vi "Read Waveform Channel(Single).vi"(7 "Timeout":i32=5000, 8 "error in (no error)":errorcluster, 11 "Waveform path in":string) -> (0 "error out":errorcluster, 2 "Waveform data":waveform(dbl), 3 "Waveform path out":string)   [LabVIEW 2019, in "DMA Channels Basic Testing.lvclass"]
uses:
  DMA Channels Basic Testing.lvclass
  <vilib>/NI VeriStand/Execution/WaveformStreaming/Set Rate for Waveform Stream (Acquisition Rate).vi
  <vilib>/NI VeriStand/Execution/WaveformStreaming/Set Condition for Waveform Stream (All Data).vi
  <vilib>/NI VeriStand/Execution/WaveformStreaming/Register for Waveform Data Events (DBL).vi
  <vilib>/NI VeriStand/Execution/WaveformStreaming/Unregister for Waveform Data Events (DBL).vi
  <vilib>/NI VeriStand/Execution/WaveformStreaming/NI_VS Waveform Streaming Interface.lvlib
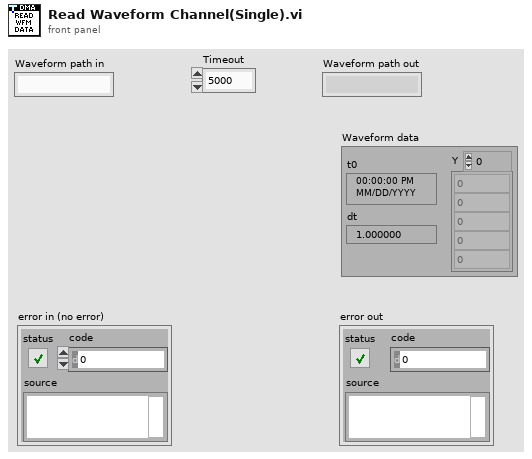
[diagram p1: front panel]
types:
  T1 = typedef "NI_VS Waveform Streaming Interface.lvlib/WaveformStreamSpecification.ctl" = refnum<k24>
  T2 = typedef "NI_VS Waveform Streaming Interface.lvlib/WaveformStreamingAPI.ctl" = refnum<k24>
  T3 = typedef "NI_VS Waveform Streaming Interface.lvlib/Registered Waveform Streams Data Event Refnum (DBL).ctl" = cluster{"Callback Refnum":refnum<k27>, "Data Event":refnum<user-event>, "Event Refnum":refnum<event-registration>, "WaveformDataWatcherDBL":T4}
  T4 = typedef "NI_VS Waveform Streaming Interface.lvlib/WaveformDataWatcherDBL.ctl" = refnum<k24>
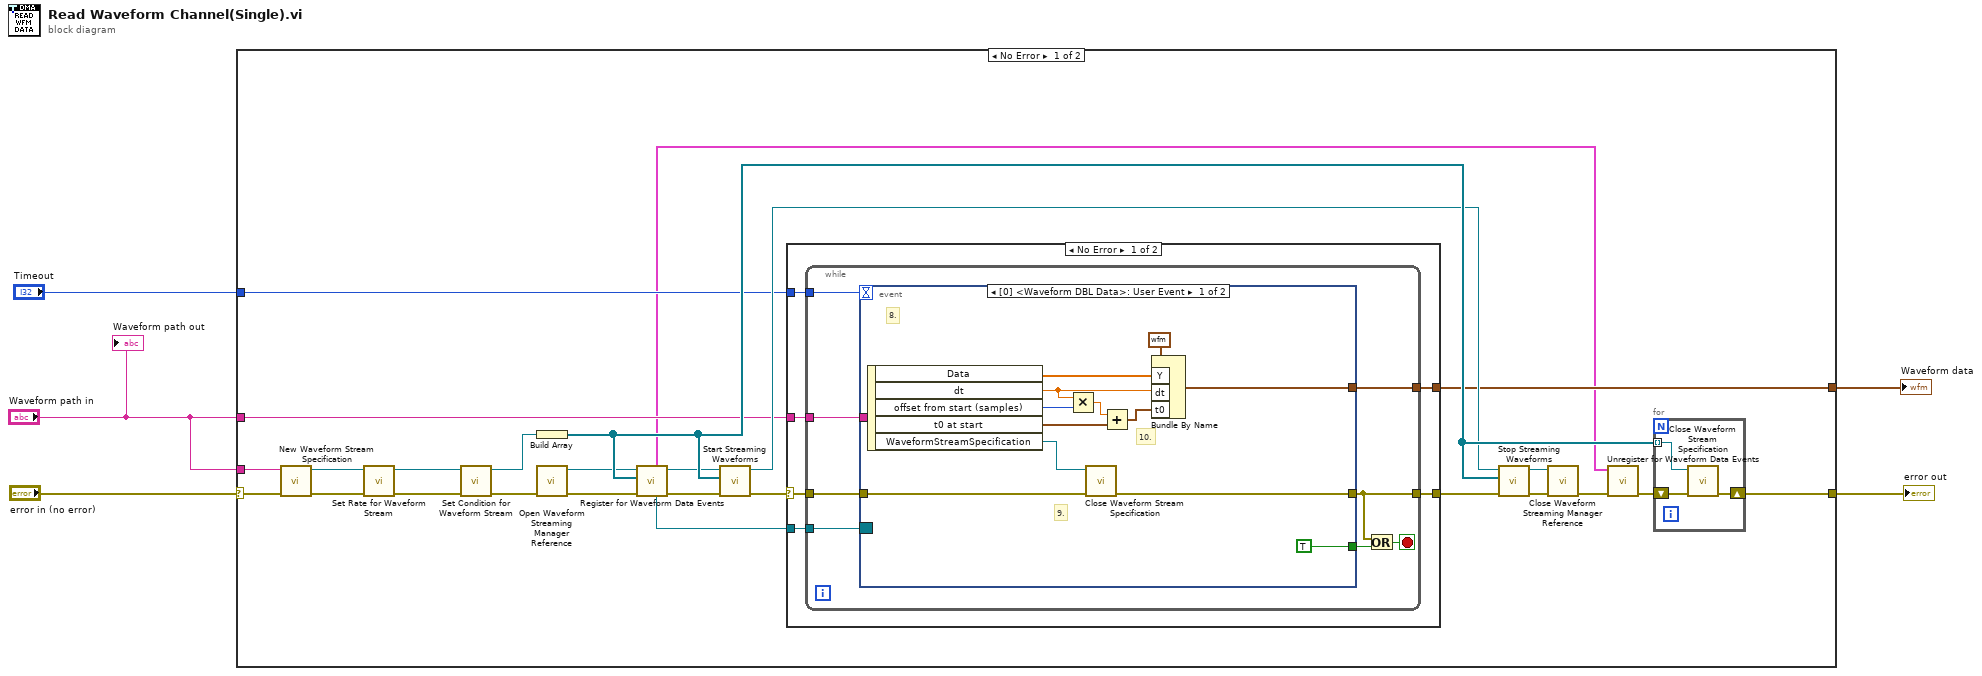
[diagram p0: block diagram]
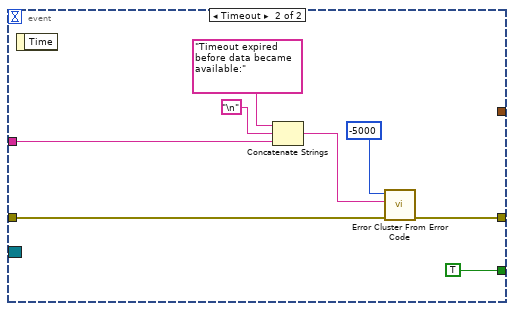
[diagram p2: hidden frame]
diagram:
  n1 = case shown="No Error" "error in (no error)" {
    selector: "error in (no error)" -> [w10 w70]
    tunnel: [w31 w70] -> w5
    tunnel: "Waveform path in" -> [w30 _]
    tunnel: [w9 _] -> w3
    tunnel: "Waveform path in" -> [w8 _]
    tunnel: "Timeout" -> [w7 _]
    frame No Error {
      n2 = call <vilib>:"New Waveform Stream Specification.vi"("error in (no error)"=w10, "waveform path"=w30) -> ("error out"=w13:errorcluster, "WaveformStreamSpecification"=w14:T1)  [unwired: 8 in]
      n3 = call-poly <vilib>:"Set Rate for Waveform Stream.vi"("error in (no error)"=w13, "WaveformStreamSpecification in"=w14) -> ("error out"=w26:errorcluster, "WaveformStreamSpecification out"=w27:T1)  [unwired: 8 in]
      n4 = call-poly <vilib>:"Set Condition for Waveform Stream.vi"("error in (no error)"=w26, "WaveformStreamSpecification in"=w27) -> ("error out"=w29:errorcluster, "WaveformStreamSpecification out"=w28:T1)  [unwired: 8 in]
      n5 = Build Array(w28) -> (w25:T1[])
      n6 = call <vilib>:"Open Waveform Streaming Manager Reference.vi"("error in (no error)"=w29) -> ("error out"=w11:errorcluster, "WaveformStreaming"=w12:T2)  [unwired: 9 in]
      n7 = call-poly <vilib>:"Register for Waveform Data Events.vi"("error in (no error)"=w11, "WaveformStreamSpecifications"=w25, "WaveformStreaming in"=w12) -> ("error out"=w15:errorcluster, "WaveformStreaming out"=w16:T2, "waveform data event registration (DBL)"=w18:refnum<event-registration>, "registered waveform data event (DBL)"=w6:T3)  [unwired: 5 in]
      n8 = call <vilib>:"Start Streaming Waveforms.vi"("error in (no error)"=w15, "WaveformStreamSpecifications"=w25, "WaveformStreaming in"=w16) -> ("error out"=w17:errorcluster, "WaveformStreaming out"=w24:T2)  [unwired: 7 in]
      n9 = case shown="No Error" w17 {
        selector: w17 -> [w40 w69]
        tunnel: [w39 w69] -> w19
        tunnel: w18 -> [w38 _]
        tunnel: [w37 _] -> w9
        tunnel: w8 -> [w36 _]
        tunnel: w7 -> [w35 _]
        frame No Error {
          n10 = while {
            tunnel: w40 -> [w47]
            tunnel: [w44] -> w39
            tunnel: w38 -> [w45]
            tunnel: [w43] -> w37
            tunnel: w36 -> [w42]
            tunnel: w35 -> [w41]
            stop <- w46 stop-if-true
            n11 = event shown="[0] <Waveform DBL Data>: User Event" {
              selector: w45 -> [_ _]
              dyn-events: _ -> [_ _]
              timeout: w41 -> [_ _]
              tunnel: [TRUE ("stop") TRUE ("stop")] -> w48
              tunnel: w47 -> [w59 w67]
              tunnel: [w52 w66] -> w44
              tunnel: [w49 _] -> w43
              tunnel: w42 -> [_ w62]
              event User Event {
                # "10."
                # "9."
                # "8."
                n12 = event-data() -> ("Data"=w50:dbl[], "dt"=w57:dbl, "offset from start (samples)"=w56:u64, "t0 at start"=w54:timestamp, "WaveformStreamSpecification"=w58:T1)  [unwired: 1 in]
                n13 = Multiply(x=w57, y=w56) -> (x*y=w55:dbl)
                n14 = call <vilib>:"Close Waveform Stream Specification.vi"("error in (no error)"=w59, "WaveformStreamSpecification"=w58) -> ("error out"=w52:errorcluster)  [unwired: 9 in]
                n15 = Add(x=w55, y=w54) -> (x+y=w53:timestamp)
                n16 = Bundle By Name(cluster=waveform(dbl) {"t0"=timestamp(0 s since 1904-01-01), "dt"=1.0, "Y"=[]} ("waveform"), "Y"=w50, "dt"=w57, "t0"=w53) -> (w49:waveform(dbl))
              }
              event Timeout {
                n17 = event-data() -> ()  [unwired: 1 in, 1 out]
                n18 = Concatenate Strings("Timeout expired before data became available:" ("error message (\"\")"), "\n", w62) -> (w61:string)
                n19 = call <vilib>:"Error Cluster From Error Code.vi"("error in (no error)"=w67, "error message (\"\")"=w61, "error code (0)"=-5000) -> ("error out"=w66:errorcluster)  [unwired: 6 in]
              }
            }
            n20 = Or(x=w44, y=w48) -> (x .or. y?=w46:bool)
          }
        }
        frame Error {
        }
      }
      n21 = call <vilib>:"Stop Streaming Waveforms.vi"("error in (no error)"=w19, "WaveformStreamSpecifications"=w25, "WaveformStreaming in"=w24) -> ("error out"=w20:errorcluster, "WaveformStreaming out"=w21:T2)  [unwired: 7 in]
      n22 = call <vilib>:"Close Waveform Streaming Manager Reference.vi"("error in (no error)"=w20, "WaveformStreaming"=w21) -> ("error out"=w22:errorcluster)  [unwired: 9 in]
      n23 = call-poly <vilib>:"Unregister for Waveform Data Events.vi"("error in (no error)"=w22, "registered waveform data event (DBL)"=w6) -> ("error out"=w23:errorcluster)  [unwired: 9 in]
      n24 = for {
        shift-right: [w33] -> w31
        shift-left: w23 -> [w34]
        tunnel: w25 -> [w32] mode=indexing
        n25 = call <vilib>:"Close Waveform Stream Specification.vi"("error in (no error)"=w34, "WaveformStreamSpecification"=w32) -> ("error out"=w33:errorcluster)  [unwired: 9 in]
      }
    }
    frame Error {
    }
  }
  "error out" <- w5
  "Waveform data" <- w3
  "Waveform path out" <- "Waveform path in"
